vi "Query Guided Calibration Kit.vi"(8 "error in (no error)":errorcluster, 10 "Connector ('Not used')":string="Not used", 11 "VISA resource name":refnum<visa-resource-name>) -> (0 "error out":errorcluster, 2 "Calibration Kits":string[](array[string]), 3 "VISA resource name out":refnum<visa-resource-name>)   [LabVIEW 2018, in "Keysight PNA Series.lvlib"]
doc: "Returns a list of valid kits that use the specified connector type."
uses:
  Keysight PNA Series.lvlib
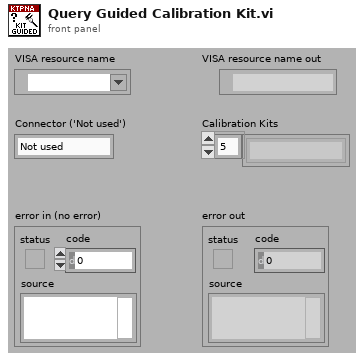
[diagram p1: front panel]
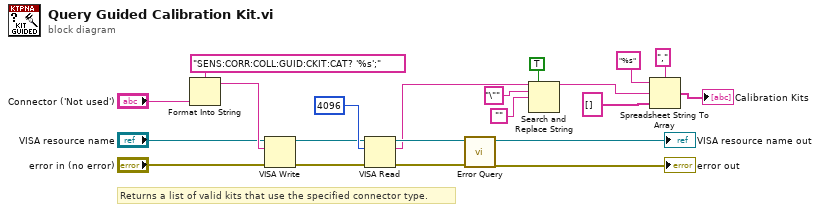
[diagram p0: block diagram]
diagram:
  # "Returns a list of valid kits that use the specified connector type."
  n1 = Format Into String(format string="SENS:CORR:COLL:GUID:CKIT:CAT? '%s';", "Connector ('Not used')") -> (resulting string=w19:string)  [unwired: 2 in, 1 out]
  n2 = VISA Write(VISA resource name="VISA resource name", write buffer=w19, error in (no error)="error in (no error)") -> (VISA resource name out=w15:refnum<visa-resource-name>, error out=w14:errorcluster)  [unwired: 1 out]
  n3 = VISA Read(VISA resource name=w15, byte count=u32 4096, error in (no error)=w14) -> (VISA resource name out=w13:refnum<visa-resource-name>, read buffer=w2:string, error out=w12:errorcluster)  [unwired: 1 out]
  n4 = call "Error Query.vi"("error in (no error)"=w12, "VISA resource name"=w13) -> ("error out"=→"error out":errorcluster, "VISA resource name out"=→"VISA resource name out":refnum<visa-resource-name>)  [unwired: 6 in, 2 out]
  n5 = Search and Replace String(replace all?=TRUE ("replace all? (F)"), input string=w2, search string="\"", replace string="") -> (result string=w3:string)  [unwired: 4 in, 3 out]
  n6 = Spreadsheet String To Array(delimiter (Tab)=",", format string="%s", spreadsheet string=w3, array type (2D Dbl)=string[] []) -> (array=→"Calibration Kits":string[])
